vi "GUID.vi"() -> (3 "trimmed string":string caption="GUID")   [LabVIEW 2020]
uses:
  Global_Variable/Global.vi
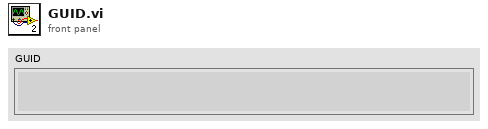
[diagram p1: front panel]
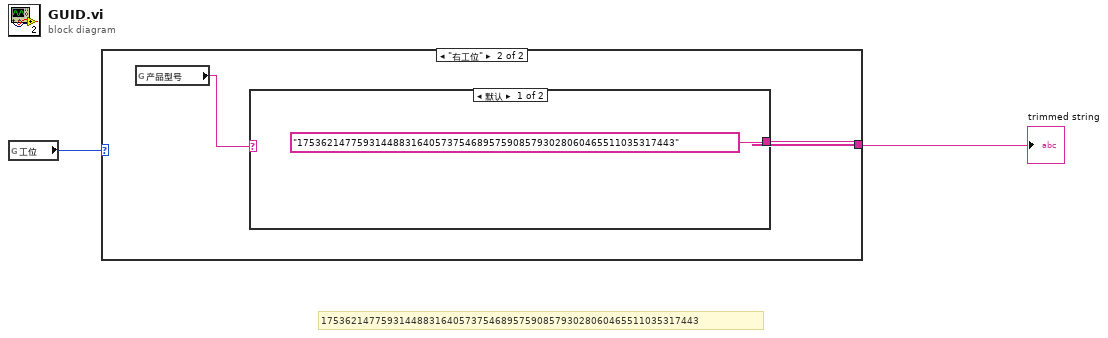
[diagram p0: block diagram]
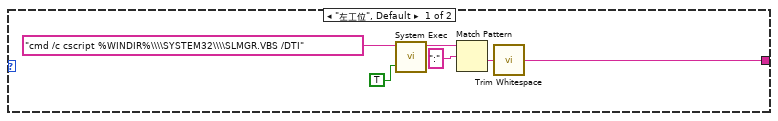
[diagram p2: hidden frame]
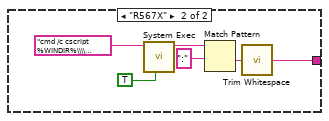
[diagram p3: hidden frame]
diagram:
  # "175362147759314488316405737546895759085793028060465511035317443"
  n1 = global read "Global.vi" "工位"() -> (w1:enum16{"左工位", "右工位"})
  n2 = case shown="\"右工位\"" w1 {
    tunnel: [w3 w10] -> w2
    frame "左工位", Default {
      n3 = call <vilib>:"System Exec.vi"("run minimized? (F)"=TRUE, "command line"="cmd /c cscript %WINDIR%\\\\SYSTEM32\\\\SLMGR.VBS /DTI") -> ("standard output"=w6:string)  [unwired: 6 in, 3 out]
      n4 = Match Pattern(string=w6, regular expression=":" ("正则表达式")) -> (after substring=w4:string)  [unwired: 1 in, 3 out]
      n5 = call <vilib>:"Trim Whitespace.vi"("string"=w4) -> ("trimmed string"=w3:string)  [unwired: 1 in]
    }
    frame "右工位" {
      n6 = global read "Global.vi" "产品型号"() -> (w9:string)
      n7 = case shown="默认" w9 {
        tunnel: ["175362147759314488316405737546895759085793028060465511035317443" w12] -> w10
        frame Default {
        }
        frame "R567X" {
          n8 = call <vilib>:"System Exec.vi"("run minimized? (F)"=TRUE, "command line"="cmd /c cscript %WINDIR%\\\\SYSTEM32\\\\SLMGR.VBS /DTI") -> ("standard output"=w17:string)  [unwired: 6 in, 3 out]
          n9 = Match Pattern(string=w17, regular expression=":" ("正则表达式")) -> (after substring=w16:string)  [unwired: 1 in, 3 out]
          n10 = call <vilib>:"Trim Whitespace.vi"("string"=w16) -> ("trimmed string"=w12:string)  [unwired: 1 in]
        }
      }
    }
  }
  "trimmed string" <- w2
